vi "csmstandapp - test run script 2.vi"() -> ()   [LabVIEW 2020, in "CSMStand(Lite)-test.lvlib"]
uses:
  CSMStand(Lite)-test.lvlib
  <userlib>/_NEVSTOP/Communicable State Machine(CSM)/Communicable State Machine.lvlib
panel:
  out "error out":errorcluster
  out "Array":cluster{string, "Response":string}[](array[cluster])
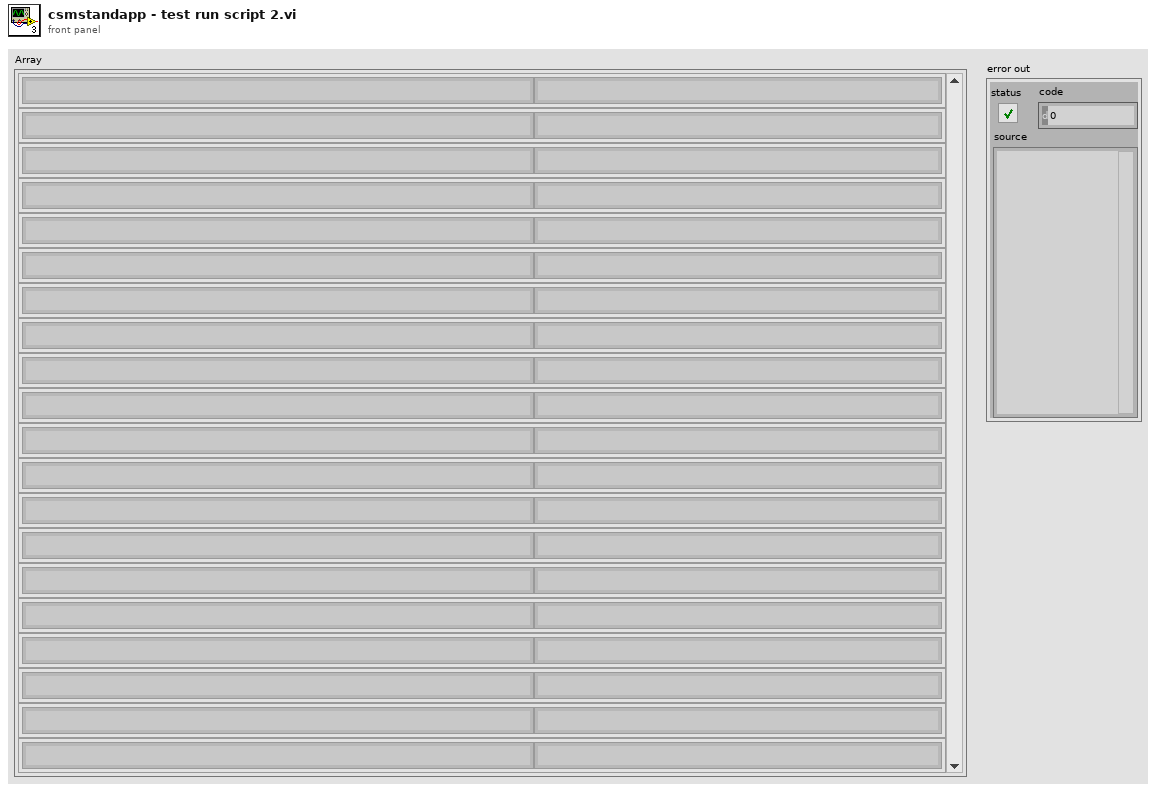
[diagram p1: front panel]
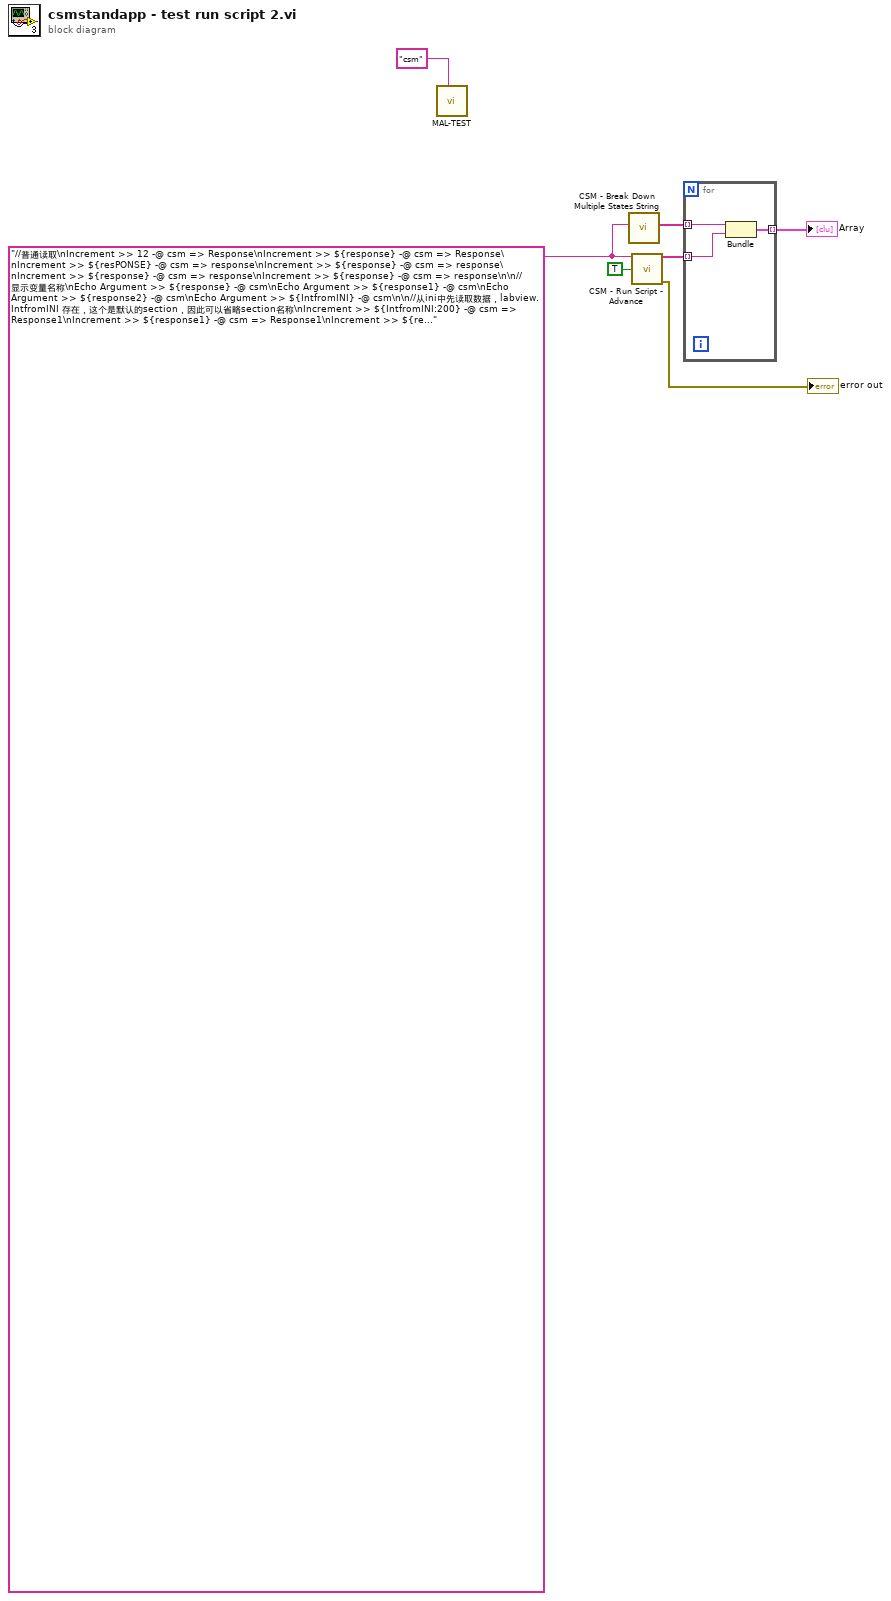
[diagram p0: block diagram]
diagram:
  w5 = "//普通读取\nIncrement >> 12 -@ csm => Response\nIncrement >> ${response} -@ csm => Response\nIncrement >> ${resPONSE} -@ csm => response\nIncrement >> ${response} -@ csm => response\nIncrement >> ${response} -@ csm => response\nIncrement >> ${response} -@ csm => response\n\n//显示变量名称\nEcho Argument >> ${response} -@ csm\nEcho Argument >> ${response1} -@ csm\nEcho Argument >> ${response2} -@ csm\nEcho Argument >> ${IntfromINI} -@ csm\n\n//从ini中先读取数据，labview.IntfromINI 存在，这个是默认的section，因此可以省略section名称\nIncrement >> ${IntfromINI:200} -@ csm => Response1\nIncrement >> ${response1} -@ csm => Response1\nIncrement >> ${resPONSE1} -@ csm => response1\nIncrement >> ${response1} -@ csm => response1\nIncrement >> ${response1} -@ csm => response1\nIncrement >> ${response1} -@ csm => response1\n\n//显示变量名称\nEcho Argument >> ${response} -@ csm\nEcho Argument >> ${response1} -@ csm\nEcho Argument >> ${response2} -@ csm\nEcho Argument >> ${IntfromINI} -@ csm\n\n//从ini中先读取数据，section.IntfromINI 不存在\nIncrement >> ${section.IntfromINI:200} -@ csm => Response2\nIncrement >> ${response2} -@ csm => Response2\nIncrement >> ${resPONSE2} -@ csm => response2\nIncrement >> ${response2} -@ csm => response2\nIncrement >> ${response2} -@ csm => response2\nIncrement >> ${response2} -@ csm => response2\n\n//显示变量名称\nEcho Argument >> ${response} -@ csm\nEcho Argument >> ${response1} -@ csm\nEcho Argument >> ${response2} -@ csm\nEcho Argument >> ${IntfromINI} -@ csm\n\n//优先从脚本创建的变量中读取数据\nIncrement >> 300 -@ csm => IntfromINI\nIncrement >> ${IntfromINI} -@ csm => IntfromINI\nIncrement >> ${IntfromINI} -@ csm => IntfromINI\nIncrement >> ${IntfromINI} -@ csm => IntfromINI\nIncrement >> ${IntfromINI} -@ csm => IntfromINI\nIncrement >> ${IntfromINI} -@ csm => IntfromINI\n\n//显示变量名称\nEcho Argument >> ${response} -@ csm\nEcho Argument >> ${response1} -@ csm\nEcho Argument >> ${response2} -@ csm\nEcho Argument >> ${IntfromINI} -@ csm\n\nRandom Cluster -@ csm => cluster\nEcho Argument >> ${cluster} -@ csm\nEcho Argument >> ${cluster.a} -@ csm\nEcho Argument >> ${cluster.b} -@ csm\nEcho Argument >> 12345 -@ csm => cluster.a\nEcho Argument >> ${cluster} -@ csm\nEcho Argument >> ${cluster.a} -@ csm\n\n\nRandom Cluster -@ csm => x;y\nEcho Argument >> ${x} -@ csm\nEcho Argument >> ${y} -@ csm\n\nRandom Array -@ csm => x;y\nEcho Argument >> ${x} -@ csm\nEcho Argument >> ${y} -@ csm\n\nRandom Array(massdata) -@ csm => x;y\nEcho Argument >> ${x} -@ csm\nEcho Argument >> ${y} -@ csm\nMacro: Exit -@ csm\n\n" ("CSM Scripts")
  n1 = call "MAL-TEST.vi"("Name(\"\" to use uuid)"="csm" ("Name(\"\" to use uuid)")) -> ()  [unwired: 11 in]
  n2 = call <userlib>:"CSM - Break Down Multiple States String.vi"("States"=w5) -> ("Multiple States"=w4:string[])  [unwired: 10 in]
  n3 = call "CSM - Run Script - Advance.vi"("CSM Scripts"=w5, "Continue If Error? (F)"=TRUE) -> ("Response"=w3:string[], "error out"=→"error out":errorcluster)  [unwired: 11 in, 1 out]
  n4 = for {
    tunnel: w4 -> [w10] mode=indexing
    tunnel: w3 -> [w9] mode=indexing
    tunnel: [w8] -> w2 mode=indexing
    n5 = Bundle(w10, "Response"=w9) -> (w8:cluster{string, "Response":string})  [unwired: 1 in]
  }
  "Array" <- w2
